vi "roller_map_user_to_output_state.vi"(11 "roller user state":T2) -> (3 "roller output state":T1)   [LabVIEW 2011]
uses:
  roller_user_state.ctl
  roller_output_state.ctl
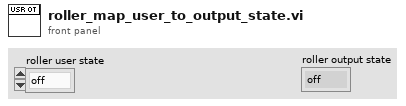
[diagram p1: front panel]
types:
  T1 = typedef "roller_output_state.ctl" = enum16{"off", "suck", "blow"}
  T2 = typedef "roller_user_state.ctl" = enum16{"off", "collect", "blow", "force suck"}
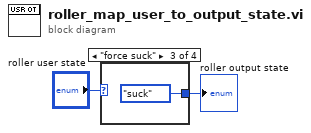
[diagram p0: block diagram]
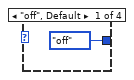
[diagram p2: hidden frame]
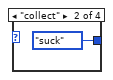
[diagram p3: hidden frame]
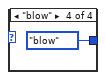
[diagram p4: hidden frame]
diagram:
  n1 = case shown="\"force suck\"" "roller user state" {
    tunnel: [roller_output_state."off" ("roller output state") roller_output_state."suck" ("roller output state") roller_output_state."suck" ("roller output state") roller_output_state."blow" ("roller output state")] -> w1
    frame "off", Default {
    }
    frame "collect" {
    }
    frame "force suck" {
    }
    frame "blow" {
    }
  }
  "roller output state" <- w1
